vi "Enqueue UI Loop.vi"(0 "UI Que In":refnum<queue>, 5 "Message":string, 7 "Test Results":T1, 11 "error in (no error)":errorcluster) -> (4 "UI Queue Out":refnum<queue>, 15 "error out":errorcluster)   [LabVIEW 2016]
doc: "This VI Enqueues a message and message data to the UI loop."
uses:
  controls/Test Results.ctl
  C:/Program Files (x86)/National Instruments/LabVIEW 2016/examples/Design Patterns/Queued Message Handler/support/QMH Fundamentals - Message Cluster.ctl
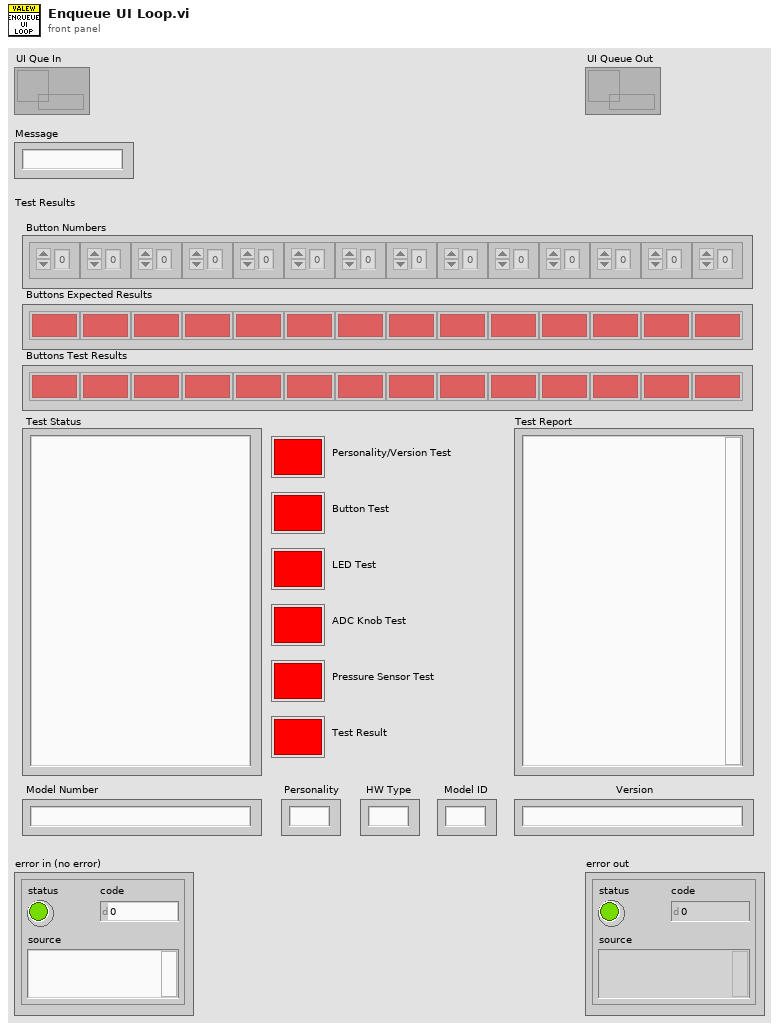
[diagram p1: front panel]
types:
  T1 = typedef "Test Results.ctl" = cluster{"Test Status":string, "Personality/Version Test ":bool, "Test Report":string, "Model Number":string, "Button Numbers":i32[], "Buttons Test Results":bool[], "Buttons Expected Results":bool[], "Model ID":string, "Personality":string, "HW Type":string, "Version":string, "Button Test":bool, "LED Test":bool, "ADC Knob Test":bool, "Pressure Sensor Test":bool, "Test Result":bool}
  T2 = typedef "QMH Fundamentals - Message Cluster.ctl" = cluster{"Message":string, "Message Data":variant}
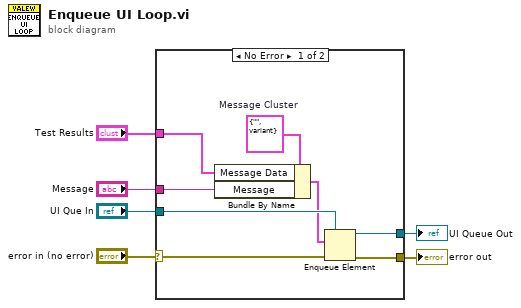
[diagram p0: block diagram]
diagram:
  n1 = case shown="No Error" "error in (no error)" {
    selector: "error in (no error)" -> [w7 w16]
    tunnel: "Test Results" -> [w14 _]
    tunnel: [w13 w16] -> w5
    tunnel: "UI Que In" -> [w12 w15]
    tunnel: "Message" -> [w11 _]
    tunnel: [w8 w15] -> w2
    frame No Error {
      w9 = T2 {"Message"="", "Message Data"=variant}  # Message Cluster
      n2 = Bundle By Name(cluster=w9, "Message Data"=w14, "Message"=w11) -> (w10:T2)
      n3 = Enqueue Element(queue=w12, element=w10, error in (no error)=w7) -> (queue out=w8:refnum<queue>, error out=w13:errorcluster)  [unwired: 1 in, 1 out]
    }
    frame Error {
    }
  }
  "error out" <- w5
  "UI Queue Out" <- w2
